vi "Savitsky Golay Filter (single).vi"(8 "error in (no error)":errorcluster, 10 "side points":i32, 11 "XY-data":cluster{"X-array":dbl[], "Y-array":dbl[]}) -> (0 "error out":errorcluster, 3 "XY-data out":cluster{"X-array":dbl[], "Y-array":dbl[]} {"Y-array" format="%.2p"; "X-array" format="%.2p"})   [LabVIEW 2019, in "xy_utilities.lvlib"]
doc: "Filter <b>XY-data</b>'s Y-Array with a Savitsky-Golay FIR smoothing filter.\n\n<b>side points</b> specifies the number of data points to each side of the current data point to use for the least squares minimization. side points*2 + 1 is the length of the moving window, which must be greater than the polynomial order.\n\nWire data to the data input to determine the polymorphic instance to use or manually select the instance."
uses:
  xy_utilities.lvlib
  <vilib>/Analysis/NI_AALBase.lvlib
  <vilib>/Analysis/3filter.llb/Savitzky-Golay Filter (DBL).vi
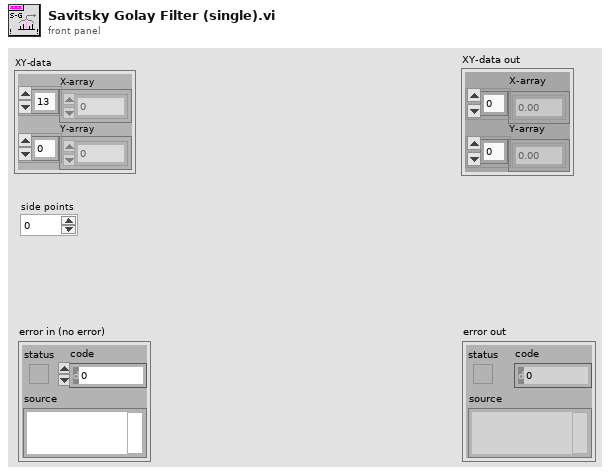
[diagram p1: front panel]
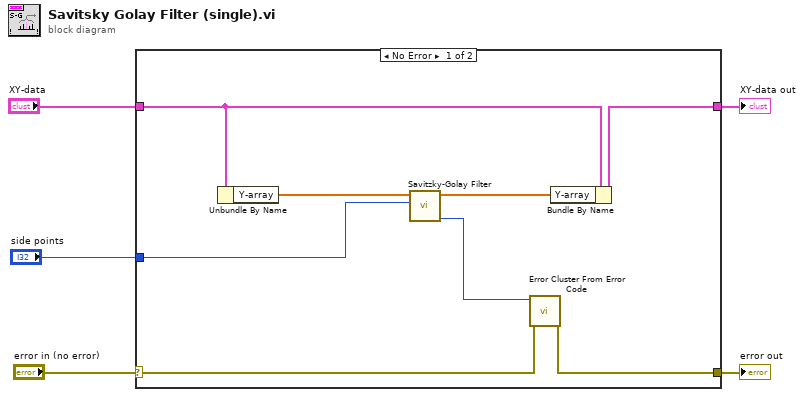
[diagram p0: block diagram]
diagram:
  n1 = case shown="No Error" "error in (no error)" {
    selector: "error in (no error)" -> [w8 w15]
    tunnel: [w7 w15] -> w4
    tunnel: "XY-data" -> [w12 w14]
    tunnel: [w13 w14] -> w2
    tunnel: "side points" -> [w6 _]
    frame No Error {
      n2 = Unbundle By Name(w12) -> ("Y-array"=w11:dbl[])
      n3 = call-poly <vilib>:"Savitzky-Golay Filter.vi"("side points"=w6, "X"=w11) -> ("error"=w9:i32, "Filtered X"=w10:dbl[])  [unwired: 8 in]
      n4 = call <vilib>:"Error Cluster From Error Code.vi"("error in (no error)"=w8, "error code (0)"=w9) -> ("error out"=w7:errorcluster)  [unwired: 7 in]
      n5 = Bundle By Name(cluster=w12, "Y-array"=w10) -> (w13:cluster{"X-array":dbl[], "Y-array":dbl[]})
    }
    frame Error {
    }
  }
  "error out" <- w4
  "XY-data out" <- w2
